vi "Extract Enum Info.vi"(11 "enum":string) -> (2 "映射表":map{u32, string}(c390), 3 "枚举名称":string)   [LabVIEW 2020]
uses:
  <vilib>/Utility/miscctls.llb/LVMapReplaceAction.ctl
  <vilib>/regexp/Match Regular Expression.xnode
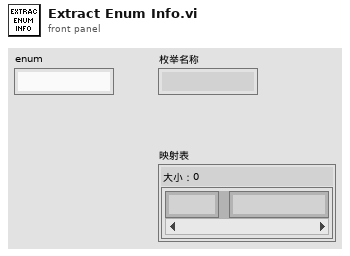
[diagram p1: front panel]
types:
  T1 = typedef "LVMapReplaceAction.ctl" = enum32{"Modify Entry only if found", "Add or Modify Entry", "Delete Entry"}
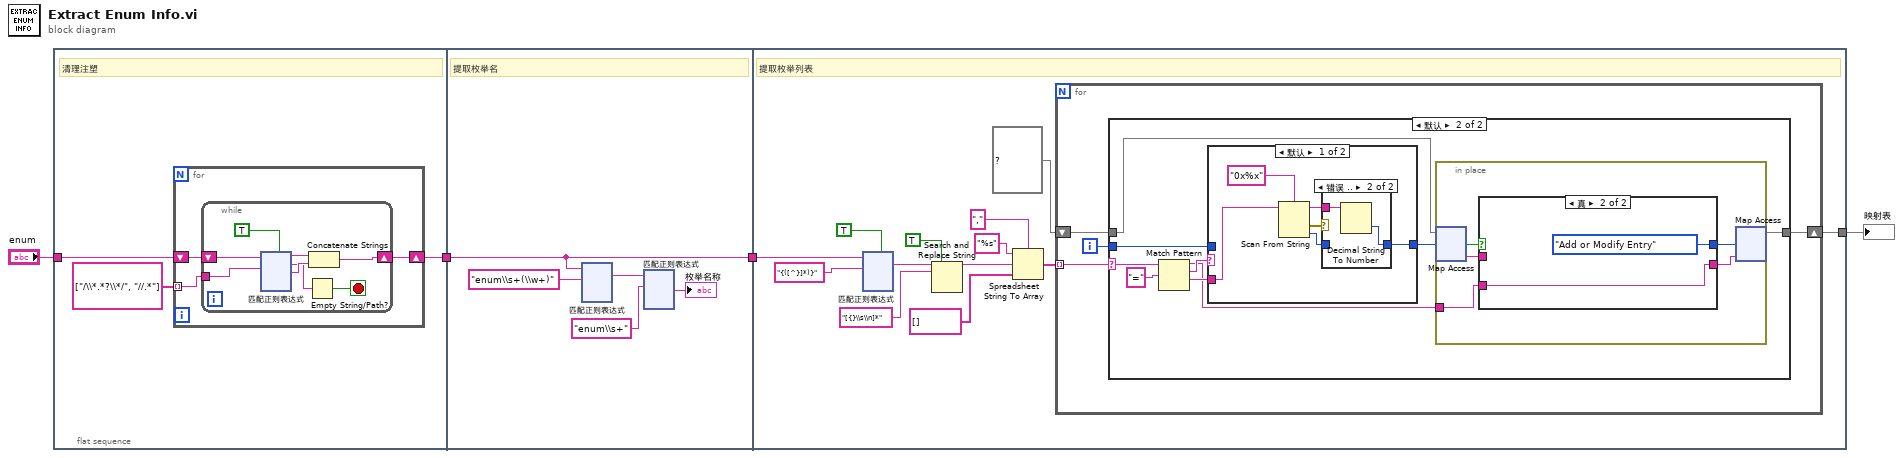
[diagram p0: block diagram]
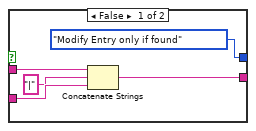
[diagram p3: hidden frame]
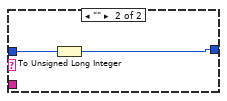
[diagram p5: hidden frame]
diagram:
  n1 = flat-sequence {
    tunnel: "enum" -> [w7]
    tunnel: [w5] -> w4
    tunnel: w4 -> [w133]
    tunnel: [w133] -> w3
    tunnel: w3 -> [w367]
    tunnel: [w366] -> w2
    frame #0 {
      # "清理注塑"
      n2 = for {
        shift-right: [w9] -> w5
        shift-left: w7 -> [w10]
        tunnel: string[] ["/\\*.*?\\*/", "//.*"] -> [w8] mode=indexing
        n3 = while {
          shift-right: [w14] -> w9
          shift-left: w10 -> [w18]
          tunnel: w8 -> [w11]
          stop <- w12 stop-if-true
          n4 = xnode "匹配正则表达式"("输入字符串"=w18, "正则表达式"=w11, "多行？<B><B>(F)</B></B>"=TRUE) -> ("匹配之前"=w16:string, "所有匹配"=w13:string, "匹配之后"=w15:string)  [unwired: 3 in, 2 out]
          n5 = Empty String/Path?(string/path=w13) -> (empty?=w12:bool)
          n6 = Concatenate Strings(w16, w15) -> (w14:string)
        }
      }
    }
    frame #1 {
      # "提取枚举名"
      n7 = xnode "匹配正则表达式"("输入字符串"=w133, "正则表达式"="enum\\s+(\\w+)") -> ("所有匹配"=w137:string)  [unwired: 4 in, 4 out]
      n8 = xnode "匹配正则表达式"("输入字符串"=w137, "正则表达式"="enum\\s+") -> ("匹配之后"=→"枚举名称":string)  [unwired: 4 in, 4 out]
    }
    frame #2 {
      # "提取枚举列表"
      n9 = xnode "匹配正则表达式"("输入字符串"=w367, "正则表达式"="{([^}]*)}", "多行？<B><B>(F)</B></B>"=TRUE) -> ("所有匹配"=w376:string)  [unwired: 3 in, 4 out]
      n10 = Search and Replace String(replace all?=TRUE ("替换全部？(F)"), input string=w376, search string="[{}\\s\\n]*" ("搜索字符串")) -> (result string=w377:string)  [unwired: 5 in, 3 out]
      n11 = Spreadsheet String To Array(delimiter (Tab)="," ("分隔符(Tab)"), format string="%s" ("格式字符串"), spreadsheet string=w377, array type (2D Dbl)=string[] []) -> (array=w378:string[])
      n12 = for {
        tunnel: w378 -> [w382] mode=indexing
        shift-right: [w379] -> w366
        shift-left: map{u32, string} {} ("映射表") -> [w380]
        i -> [w381]
        n13 = case shown="默认" w382 {
          selector: w382 -> [_ w392]
          tunnel: w381 -> [_ w388]
          tunnel: w380 -> [w383 w387]
          tunnel: [w383 w386] -> w379
          frame "" {
          }
          frame Default {
            n14 = Match Pattern(string=w392, regular expression="=" ("正则表达式")) -> (before substring=w384:string, match substring=w389:string, after substring=w390:string)  [unwired: 1 in, 1 out]
            n15 = case shown="默认" w389 {
              tunnel: w390 -> [w410 _]
              tunnel: [w405 w414] -> w385
              tunnel: w388 -> [_ w415]
              frame Default {
                n16 = Scan From String(format string="0x%x" ("格式字符串"), input string=w410) -> (remaining string=w407:string, error out=w408:errorcluster, output 1=w406:u32)  [unwired: 3 in, 1 out]
                n17 = case shown="错误 .." w408 {
                  tunnel: w407 -> [_ w413]
                  tunnel: w406 -> [w411 _]
                  tunnel: [w411 w412] -> w405
                  frame No Error {
                  }
                  frame Error {
                    n18 = Decimal String To Number(string=w413) -> (number=w412:i32)  [unwired: 2 in, 1 out]
                  }
                }
              }
              frame "" {
                n19 = To Unsigned Long Integer(number=w415) -> (unsigned 32bit integer=w414:u32)
              }
            }
            n20 = in-place {
              in-place-border: w384 -> [w393]
              n21 = in-place-map #1(w387, w385) -> (w396:string, w397:bool)  [unwired: 1 in]
              n22 = case shown="真" w397 {
                tunnel: w396 -> [w401 _]
                tunnel: [w398 w403] -> w395
                tunnel: [LVMapReplaceAction."Modify Entry only if found" ("操作") LVMapReplaceAction."Add or Modify Entry" ("操作")] -> w394
                tunnel: w393 -> [w400 w403]
                frame False {
                  n23 = Concatenate Strings(w401, "|" ("字符串"), w400) -> (w398:string)
                }
                frame True {
                }
              }
              n24 = in-place-map #1(w395, w394) -> (w386:map{u32, string})  [unwired: 2 out]
            }
          }
        }
      }
    }
  }
  "映射表" <- w2
